vi "Write TX Timestamp.vi"(8 "error in (no error)":errorcluster, 10 "TX Timestamp":timestamp, 11 "MB_ADU_Serial in":refnum<class "MB_ADU.lvclass">) -> (0 "error out":errorcluster, 3 "MB_ADU_Serial out":refnum<class "MB_ADU.lvclass">)   [LabVIEW 2012, in "MB Master.lvlib" / "MB_ADU.lvclass"]
uses:
  MB_ADU.lvclass
  MB_ADU.lvclass/MB_ADU.ctl
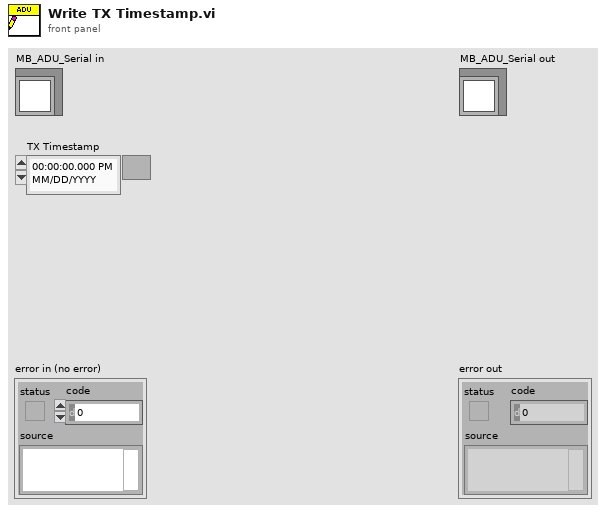
[diagram p1: front panel]
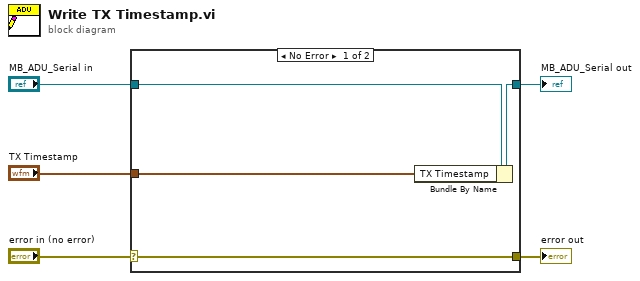
[diagram p0: block diagram]
diagram:
  n1 = case shown="No Error" "error in (no error)" {
    selector: "error in (no error)" -> [w9 w10]
    tunnel: [w9 w10] -> w4
    tunnel: [w7 w11] -> w2
    tunnel: "MB_ADU_Serial in" -> [w8 w11]
    tunnel: "TX Timestamp" -> [w6 _]
    frame No Error {
      n2 = Bundle By Name(cluster=w8, "TX Timestamp"=w6) -> (w7:refnum<class "MB_ADU.lvclass">)
    }
    frame Error {
    }
  }
  "error out" <- w4
  "MB_ADU_Serial out" <- w2
